vi "Read Waveform Measurement (Px).vi"(0 "VISA resource name":refnum<visa-resource-name>, 5 "Parameter (0: P1)":u16(ring) items=["P1", "P2", "P3", "P4", "P5", "P6", "P7", "P8"], 11 "error in (no error)":errorcluster) -> (4 "VISA resource name out":refnum<visa-resource-name>, 6 "Value":dbl format="%#_6e", 8 "Status":string, 15 "error out":errorcluster)   [LabVIEW 2013, in "LeCroy Wave Series.lvlib"]
doc: "This VI reads a the result of the parameter measured on P1 through P8 and returns the status. Note that for multi-valued parameters (parameters that can return more than 1 value per sweep) the value is the last measured event, and not the average over the entire waveform. \n\nAvailable parameters is model dependant - most models support reading back P1-P5. Attempting to read back a non-existent parameter will result in an unresolved parsing error from the instrument."
uses:
  LeCroy Wave Series.lvlib
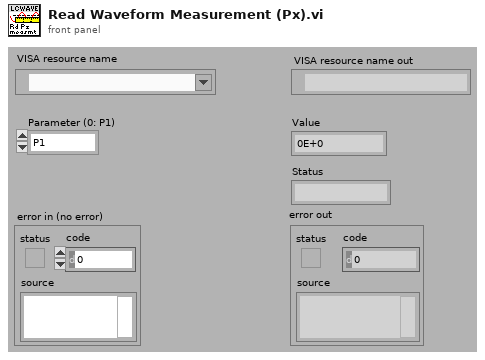
[diagram p1: front panel]
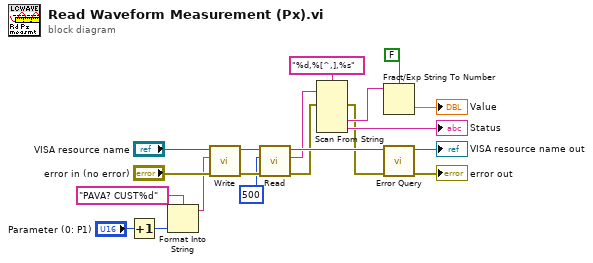
[diagram p0: block diagram]
diagram:
  n1 = Increment(x="Parameter (0: P1)") -> (x+1=w8:u16)
  n2 = Format Into String(format string="PAVA? CUST%d", w8) -> (resulting string=w11:string)  [unwired: 2 in, 1 out]
  n3 = call "Write.vi"("error in (no error)"="error in (no error)", "Write Buffer"=w11, "VISA resource name"="VISA resource name") -> ("error out"=w16:errorcluster, "VISA resource name out"=w17:refnum<visa-resource-name>)  [unwired: 6 in, 1 out]
  n4 = call "Read.vi"("error in (no error)"=w16, "Byte Count"=u32 500, "VISA resource name"=w17) -> ("error out"=w3:errorcluster, "Read Buffer"=w6:string, "VISA resource name out"=w14:refnum<visa-resource-name>)  [unwired: 5 in, 1 out]
  n5 = Scan From String(format string="%d,%[^,],%s", input string=w6, error in=w3) -> (error out=w2:errorcluster, output 2=w5:string, output 3=→"Status":string)  [unwired: 5 in, 2 out]
  n6 = Fract/Exp String To Number(use system decimal point (T)=FALSE, string=w5) -> (number=→"Value":dbl)  [unwired: 2 in, 1 out]
  n7 = call "Error Query.vi"("error in (no error)"=w2, "VISA resource name"=w14) -> ("error out"=→"error out":errorcluster, "VISA resource name out"=→"VISA resource name out":refnum<visa-resource-name>)  [unwired: 6 in, 2 out]
